vi "MoveToXYZ.vi"(7 "MM System":u16(ring) items=["MM3000", "MM2000"]) -> ()   [LabVIEW 2022 SP3]
uses:
  -MotionRoutines/MotionGlobals.vi
  -Mm2000/MM2000 Position Absolute Wait.vi
panel:
  in  "ExitSendCmd":bool
  in  "Z reset":bool
  in  "Z axis":dbl format="%.3f"
  in  "Y reset":bool
  in  "Y Axis":dbl format="%.3f"
  in  "X reset":bool
  in  "X Axis":dbl format="%.3f"
  # "Units are in cm.\n\"Rst\" zeros the position"
  # "X Axis"
  # "Y Axis"
  # "Z Axis"
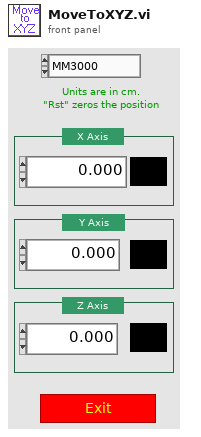
[diagram p1: front panel]
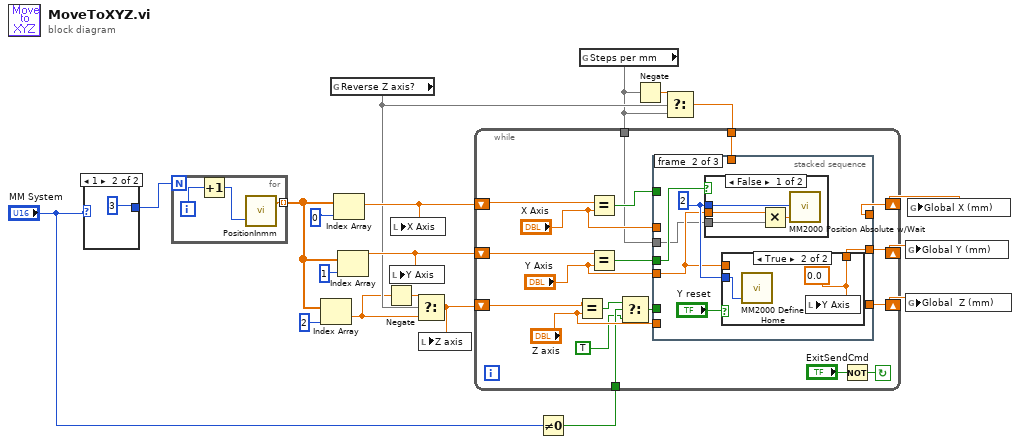
[diagram p0: block diagram]
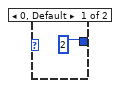
[diagram p2: hidden frame]
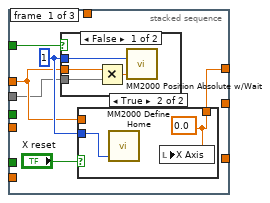
[diagram p3: hidden frame]
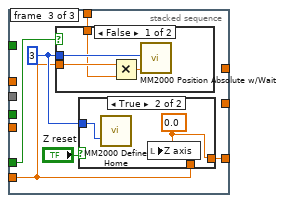
[diagram p8: hidden frame]
diagram:
  n1 = case shown="1" "MM System" {
    tunnel: [2 3] -> w4
    frame 0, Default {
    }
    frame 1 {
    }
  }
  n2 = for {
    N: w4 -> [_]
    tunnel: [w22] -> w15 mode=indexing
    i -> [w24]
    n3 = Increment(x=w24) -> (x+1=w23:i32)
    n4 = call "PositionInmm.vi"("Axis"=w23) -> ("postion in mm"=w22:dbl)  [unwired: 1 in, 1 out]
  }
  n5 = Index Array(array=w15, index=2 ("Axis")) -> (element=w6:dbl)
  n6 = global read "MotionGlobals.vi" "Reverse Z axis?"() -> (w8)
  n7 = Index Array(array=w15, index=0 ("Index")) -> (element=w12:dbl)
  n8 = Index Array(array=w15, index=1 ("Axis")) -> (element=w11:dbl)
  n9 = Negate(x=w6) -> (-x=w7:dbl)
  n10 = local write "Y Axis"(w11) -> ()
  n11 = local write "X Axis"(w12) -> ()
  n12 = Select(t=w7, s=w8, f=w6) -> (s? t:f=w5:dbl)
  n13 = local write "Z axis"(w5) -> ()
  n14 = Not Equal To 0?(x="MM System") -> (x != 0?=w1:bool)
  n15 = global read "MotionGlobals.vi" "Steps per mm"() -> (w2)
  n16 = Negate(x=w2) -> (-x=w10:dbl)
  n17 = Select(t=w10, s=w8, f=w2) -> (s? t:f=w9:dbl)
  n18 = while {
    tunnel: w9 -> [w30]
    shift-left: w5 -> [w43]
    shift-right: [w31] -> w17
    shift-left: w11 -> [w42]
    shift-right: [w35] -> w18
    shift-left: w12 -> [w41]
    shift-right: [w36] -> w19
    tunnel: w2 -> [w29]
    tunnel: w1 -> [w26]
    stop <- w37 continue-if-true
    n19 = Equal?(x=w43, y="Z axis") -> (x = y?=w27:bool)
    n20 = Equal?(x=w41, y="X Axis") -> (x = y?=w40:bool)
    n21 = Equal?(x=w42, y="Y Axis") -> (x = y?=w39:bool)
    n22 = Select(t=w27, s=w26, f=TRUE) -> (s? t:f=w28:bool)
    n23 = stacked-sequence {
      tunnel: w40 -> [w48 _ _]
      tunnel: w39 -> [_ w60 _]
      tunnel: w28 -> [_ _ w73]
      tunnel: "X Axis" -> [w45 _ _]
      tunnel: "Y Axis" -> [_ w59 _]
      tunnel: "Z axis" -> [_ _ w72]
      tunnel: [w46 _ _] -> w36
      tunnel: [_ w58 _] -> w35
      tunnel: [_ _ w71] -> w31
      tunnel: w30 -> [_ _ w70]
      tunnel: w29 -> [w44 w57 _]
      frame #0 {
        w47 = 1 ("Axis")
        n24 = case shown="False" w48 {
          tunnel: w47 -> [w52 _]
          tunnel: w45 -> [w51 _]
          tunnel: w44 -> [w50 _]
          frame False {
            n25 = Multiply(x=w51, y=w50) -> (x*y=w53:dbl)
            n26 = call "MM2000 Position Absolute w/Wait.vi"("Position Absolute"=w53, "Axis"=w52) -> ()  [unwired: 1 in]
          }
          frame True {
          }
        }
        n27 = case shown="True" "X reset" {
          tunnel: w47 -> [_ w56]
          tunnel: [w54 w55] -> w46
          tunnel: w45 -> [w54 _]
          frame False {
          }
          frame True {
            w55 = 0.0 ("Z axis")
            n28 = call "MM2000 Define Home.vi"("Axis"=w56) -> ()  [unwired: 1 in]
            n29 = local write "X Axis"(w55) -> ()
          }
        }
      }
      frame #1 {
        w61 = 2 ("Axis")
        n30 = case shown="False" w60 {
          tunnel: w61 -> [w65 _]
          tunnel: w59 -> [w64 _]
          tunnel: w57 -> [w63 _]
          frame False {
            n31 = Multiply(x=w64, y=w63) -> (x*y=w66:dbl)
            n32 = call "MM2000 Position Absolute w/Wait.vi"("Position Absolute"=w66, "Axis"=w65) -> ()  [unwired: 1 in]
          }
          frame True {
          }
        }
        n33 = case shown="True" "Y reset" {
          tunnel: w61 -> [_ w69]
          tunnel: w59 -> [w67 _]
          tunnel: [w67 w68] -> w58
          frame False {
          }
          frame True {
            w68 = 0.0 ("Y Axis")
            n34 = call "MM2000 Define Home.vi"("Axis"=w69) -> ()  [unwired: 1 in]
            n35 = local write "Y Axis"(w68) -> ()
          }
        }
      }
      frame #2 {
        w74 = 3 ("Axis")
        n36 = case shown="False" w73 {
          tunnel: w74 -> [w79 _]
          tunnel: w72 -> [w78 _]
          tunnel: w70 -> [w76 _]
          frame False {
            n37 = Multiply(x=w78, y=w76) -> (x*y=w77:dbl)
            n38 = call "MM2000 Position Absolute w/Wait.vi"("Position Absolute"=w77, "Axis"=w79) -> ()  [unwired: 1 in]
          }
          frame True {
          }
        }
        n39 = case shown="True" "Z reset" {
          tunnel: w74 -> [_ w82]
          tunnel: [w80 w81] -> w71
          tunnel: w72 -> [w80 _]
          frame False {
          }
          frame True {
            w81 = 0.0 ("X Axis")
            n40 = call "MM2000 Define Home.vi"("Axis"=w82) -> ()  [unwired: 1 in]
            n41 = local write "Z axis"(w81) -> ()
          }
        }
      }
    }
    n42 = Not(x="ExitSendCmd") -> (.not. x?=w37:bool)
  }
  n43 = global write "MotionGlobals.vi" "Global Y (mm)"(w18) -> ()
  n44 = global write "MotionGlobals.vi" "Global  Z (mm)"(w17) -> ()
  n45 = global write "MotionGlobals.vi" "Global X (mm)"(w19) -> ()
